vi "Count Atoms in Structure.vi"(11 "Structure":T2) -> (3 "Atom Counts":T1(array[cluster]))   [LabVIEW 2010]
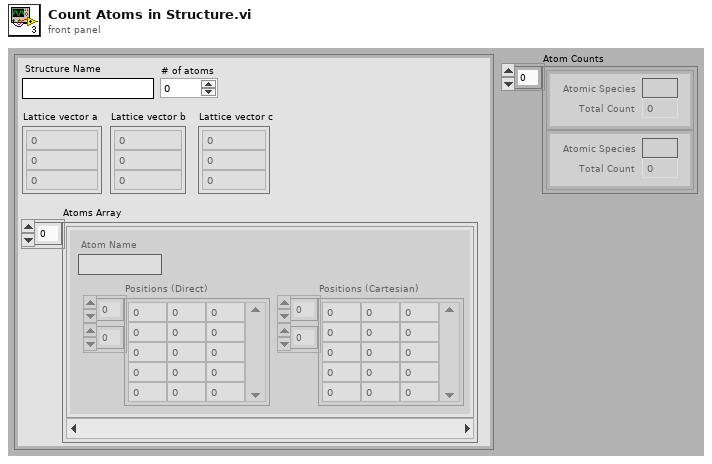
[diagram p1: front panel]
types:
  T1 = cluster{"Atomic Species":string, "Total Count":i32}[]
  T2 = cluster{"Structure Name":string, "Lattice vector a":dbl[], "Lattice vector b":dbl[], "Lattice vector c":dbl[], "Atoms Array":cluster{"Atom Name":string, "Positions (Direct)":dbl[][], "Positions (Cartesian)":dbl[][]}[], "# of atoms":i32}
  T3 = cluster{"Atom Name":string, "Positions (Direct)":dbl[][], "Positions (Cartesian)":dbl[][]}[]
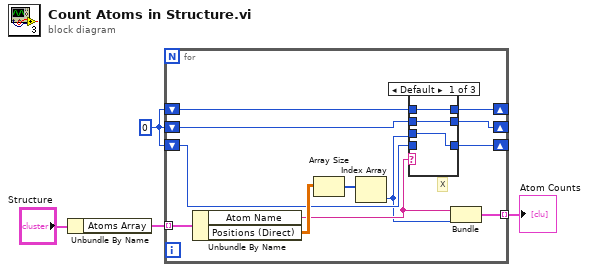
[diagram p0: block diagram]
diagram:
  w2 = 0
  n1 = Unbundle By Name("Structure") -> ("Atoms Array"=w4:T3)
  n2 = for {
    tunnel: w4 -> [w16] mode=indexing
    shift-right: [w13] -> _
    shift-left: w2 -> [w11]
    shift-right: [w12] -> _
    shift-left: w2 -> [w10]
    shift-right: [w9] -> _
    shift-left: w2 -> [w8]
    tunnel: [w5] -> w1 mode=indexing
    # "X"
    n3 = Unbundle By Name(w16) -> ("Atom Name"=w7:string, "Positions (Direct)"=w15:dbl[][])
    n4 = Array Size(array=w15) -> (size(s)=w14:i32[])
    n5 = Index Array(array=w14) -> (element=w6:i32)  [unwired: 1 in]
    n6 = case shown="Default" w7 {
      tunnel: [w18 w22 w24] -> w13
      tunnel: w6 -> [w19 w22 w25]
      tunnel: [w17 w21 w25] -> w12
      tunnel: w11 -> [w18 _ w24]
      tunnel: w10 -> [w17 w21 _]
      tunnel: [w19 w20 w23] -> w9
      tunnel: w8 -> [_ w20 w23]
      frame Default {
      }
      frame "Cd" {
      }
      frame "Te" {
      }
    }
    n7 = Bundle("Atom Name"=w7, w6) -> (w5:cluster{"Atom Name":string, i32})  [unwired: 1 in]
  }
  "Atom Counts" <- w1
